vi "Query.vi"(8 "error in (no error)":errorcluster, 10 "Query":string, 11 "Module ID":i32=-1) -> (0 "error out":errorcluster, 2 "Reply Payload":T1={"Return Data"=[], "Meta Data"=variant(cluster{"Affected Rows":u64, "Insert ID":u64, "Server Status":u16, "Warning Count":u16, "Message":string} {"Affected Rows"=0, "Insert ID"=0, "Server Status"=0, "Warning Count"=0, "Message"=""}), "Field Names"=[], "Query_error"={"status"=FALSE, "code"=0, "source"=""}})   [LabVIEW 2014, in "DB_CONNECTOR.lvlib"]
doc: "Send a SQL-Query to the database.\n_____\nCreated using Delacor QMH Event Scripter 4.0.0.57.\n\n<b>Note:</b> This VI was modified by the <b>Validate DQMH Module</b> tool to return an error if the reply times out."
uses:
  DB_CONNECTOR.lvlib
  Query (Reply Payload)--cluster.ctl
  Query Argument--cluster.ctl
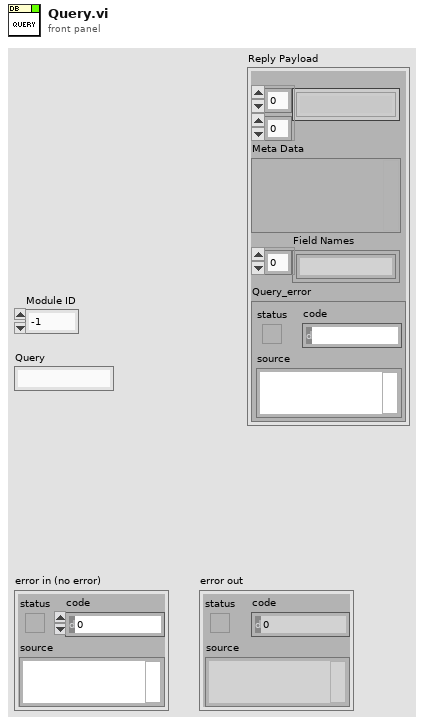
[diagram p1: front panel]
types:
  T1 = typedef "DB_CONNECTOR.lvlib/Query (Reply Payload)--cluster.ctl" = cluster{"Return Data":string[][], "Meta Data":variant, "Field Names":string[], "Query_error":errorcluster}
  T2 = typedef "DB_CONNECTOR.lvlib/Query Argument--cluster.ctl" = cluster{"Module ID":i32, "Query":string, "Wait Notifier":refnum<notifier>}
  T3 = typedef "DB_CONNECTOR.lvlib/Request Events--cluster.ctl" = cluster{"Stop Module":refnum<user-event>, "Show Panel":refnum<user-event>, "Hide Panel":refnum<user-event>, "Show Diagram":refnum<user-event>, "Get Module Execution Status":refnum<user-event>, "Configure":refnum<user-event>, "Connect":refnum<user-event>, "Query":refnum<user-event>, "Close Connection":refnum<user-event>, "Start Transaction":refnum<user-event>, "Commit Transaction":refnum<user-event>, "Fast Query":refnum<user-event>, "Get DB-Type":refnum<user-event>}
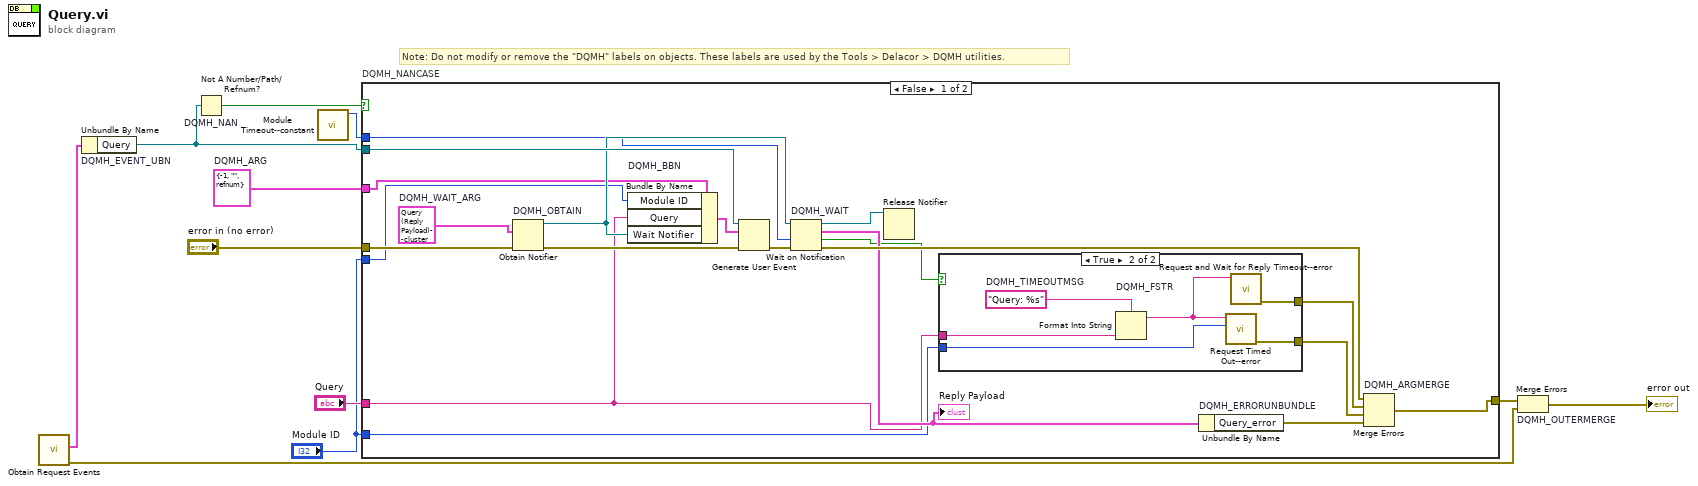
[diagram p0: block diagram]
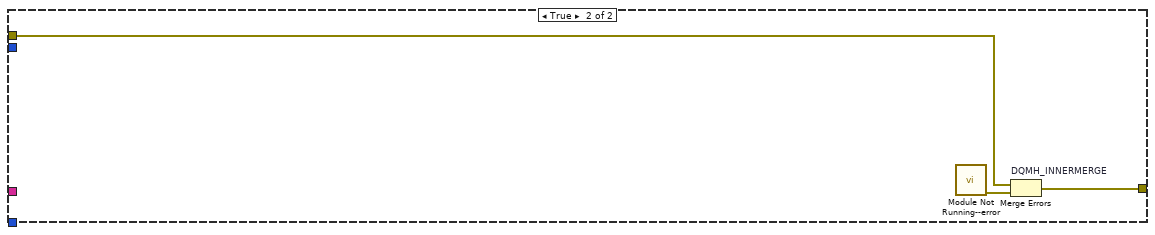
[diagram p3: hidden frame]
diagram:
  w6 = T2 {"Module ID"=-1, "Query"="", "Wait Notifier"=refnum}  # DQMH_ARG
  # "Note: Do not modify or remove the \"DQMH\" labels on objects. These labels are used by the Tools > Delacor > DQMH utilities."
  n1 = call "Obtain Request Events.vi"() -> ("error out"=w2:errorcluster, "DB_CONNECTOR Request Events"=w1:T3)  [unwired: 10 in]
  n2 = Unbundle By Name "DQMH_EVENT_UBN"(w1) -> ("Query"=w9:refnum<user-event>)
  n3 = Not A Number/Path/Refnum? "DQMH_NAN"(number/path/refnum=w9) -> (NaN/Path/Refnum?=w8:bool)
  n4 = call "Module Timeout--constant.vi"() -> ("Module Timeout"=w4:i32)  [unwired: 11 in]
  n5 = case "DQMH_NANCASE" shown="False" w8 {
    tunnel: "error in (no error)" -> [w31 w40]
    tunnel: w9 -> [w29 _]
    tunnel: [w16 w39] -> w7
    tunnel: w6 -> [w21 _]
    tunnel: "Module ID" -> [w20 _]
    tunnel: "Query" -> [w13 _]
    tunnel: w4 -> [w19 _]
    tunnel: "Module ID" -> [w18 _]
    frame False {
      w27 = T1 {"Return Data"=[], "Meta Data"=variant(cluster{"Affected Rows":u64, "Insert ID":u64, "Server Status":u16, "Warning Count":u16, "Message":string} {"Affected Rows"=0, "Insert ID"=0, "Server Status"=0, "Warning Count"=0, "Message"=""}), "Field Names"=[], "Query_error"={"status"=FALSE, "code"=0, "source"=""}}  # DQMH_WAIT_ARG
      n6 = Obtain Notifier "DQMH_OBTAIN"(notification data type=w27, error in (no error)=w31) -> (notifier out=w25:refnum<notifier>, error out=w28:errorcluster)  [unwired: 2 in, 1 out]
      n7 = Bundle By Name "DQMH_BBN"(cluster=w21, "Module ID"=w20, "Query"=w13, "Wait Notifier"=w25) -> (w22:T2)
      n8 = Generate User Event(user event=w29, event data cluster=w22, error in=w28) -> (error out=w30:errorcluster)  [unwired: 1 in, 1 out]
      n9 = Wait on Notification "DQMH_WAIT"(notifier=w25, timeout in ms (-1)=w19, error in (no error)=w30) -> (notifier out=w24:refnum<notifier>, notification=w23:T1, timed out?=w17:bool, error out=w26:errorcluster)  [unwired: 1 in]
      "Reply Payload" <- w23
      n10 = Release Notifier(notifier=w24) -> ()  [unwired: 2 in, 3 out]
      n11 = case shown="True" w17 {
        tunnel: w18 -> [_ w36]
        tunnel: [_ w34] -> w14
        tunnel: w13 -> [_ w33]
        tunnel: [_ w32] -> w12
        frame False {
        }
        frame True {
          w37 = "Query: %s"  # DQMH_TIMEOUTMSG
          n12 = Format Into String "DQMH_FSTR"(format string=w37, w33) -> (resulting string=w35:string)  [unwired: 2 in, 1 out]
          n13 = call "Request Timed Out--error.vi"("Module ID"=w36, "Request"=w35) -> ("error out"=w34:errorcluster)  [unwired: 9 in]
          n14 = call "Request and Wait for Reply Timeout--error.vi"("Error Message"=w35) -> ("error out"=w32:errorcluster)  [unwired: 10 in]
        }
      }
      n15 = Unbundle By Name "DQMH_ERRORUNBUNDLE"(w23) -> ("Query_error"=w15:errorcluster)
      n16 = Merge Errors "DQMH_ARGMERGE"(w26, w12, w14, w15) -> (w16:errorcluster)
    }
    frame True {
      n17 = call "Module Not Running--error.vi"() -> ("error out"=w38:errorcluster)  [unwired: 11 in]
      n18 = Merge Errors "DQMH_INNERMERGE"(w40, w38) -> (w39:errorcluster)
    }
  }
  n19 = Merge Errors "DQMH_OUTERMERGE"(w7, w2) -> (→"error out":errorcluster)
